vi "ukol1.vi"() -> ()   [LabVIEW 2023]
uses:
  <vilib>/Analysis/2dsp.llb/1D Convolution (DBL).vi
  <vilib>/Analysis/NI_AALPro.lvlib
panel:
  in  "Array 7":dbl[](array[numeric])
  in  "Array 6":dbl[](array[numeric])
  out "Waveform Graph":dbl[][](graph)
  in  "Array 4":dbl[](array[numeric])
  in  "Array 3":dbl[](array[numeric])
  out "X * Y":dbl[](array[numeric])
  out "Array 2":dbl[](array[numeric])
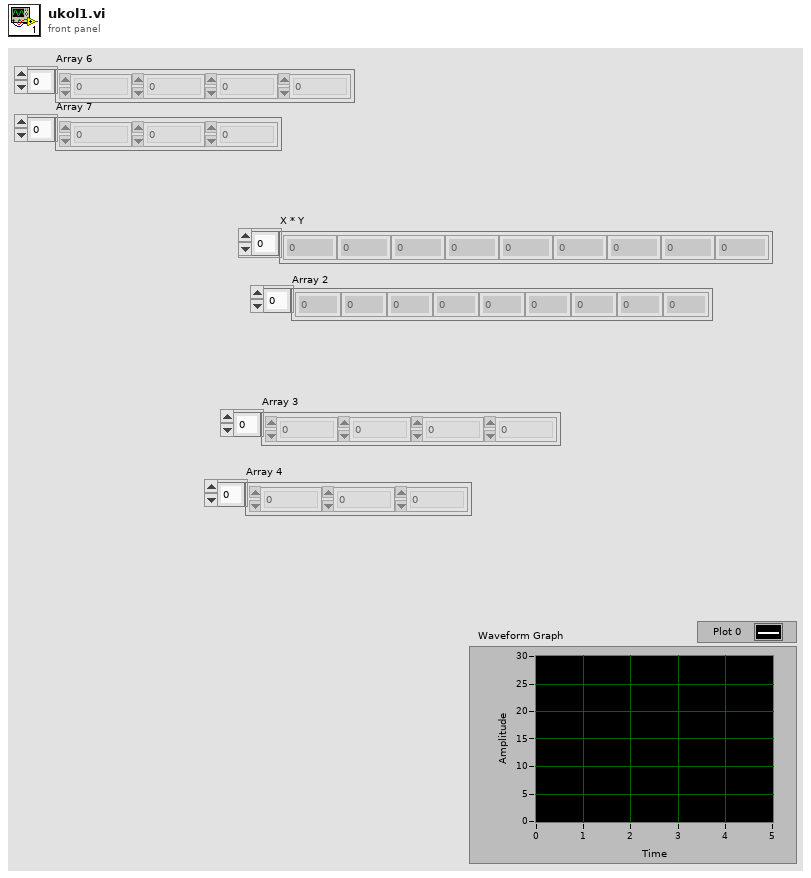
[diagram p1: front panel]
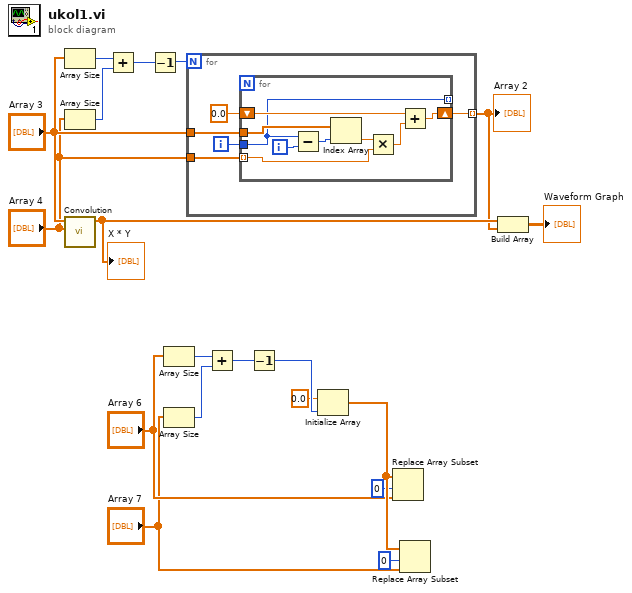
[diagram p0: block diagram]
diagram:
  n1 = Array Size(array="Array 3") -> (size(s)=w18:i32)
  n2 = Array Size(array="Array 4") -> (size(s)=w17:i32)
  n3 = call-poly <vilib>:"Convolution.vi"("Y"="Array 4", "X"="Array 3") -> ("X * Y"=w13:dbl[])  [unwired: 8 in, 1 out]
  "X * Y" <- w13
  n4 = Add(x=w18, y=w17) -> (x+y=w19:i32)
  n5 = Decrement(x=w19) -> (x-1=w16:i32)
  n6 = Array Size(array="Array 6") -> (size(s)=w9:i32)
  n7 = Array Size(array="Array 7") -> (size(s)=w8:i32)
  n8 = for {
    N: w16 -> [_]
    tunnel: "Array 3" -> [w20]
    tunnel: "Array 4" -> [w23]
    tunnel: [w22] -> w12 mode=indexing
    i -> [w21]
    n9 = for {
      shift-right: [w31] -> w22
      shift-left: 0.0 -> [w32]
      tunnel: w23 -> [w30] mode=indexing
      tunnel: w21 -> [w25]
      tunnel: w20 -> [w28]
      tunnel: [w25] -> _ mode=indexing
      i -> [w29]
      n10 = Subtract(x=w25, y=w29) -> (x-y=w27:i32)
      n11 = Index Array(array=w28, index=w27) -> (element=w26:dbl)
      n12 = Multiply(x=w26, y=w30) -> (x*y=w33:dbl)
      n13 = Add(x=w32, y=w33) -> (x+y=w31:dbl)
    }
  }
  "Array 2" <- w12
  n14 = Add(x=w9, y=w8) -> (x+y=w10:i32)
  n15 = Decrement(x=w10) -> (x-1=w7:i32)
  n16 = Initialize Array(0.0 ("element"), w7) -> (w5:dbl[])
  n17 = Replace Array Subset(array=w5, new element="Array 6", index=0) -> ()  [unwired: 1 out]
  n18 = Replace Array Subset(array=w5, new element="Array 7", index=0) -> ()  [unwired: 1 out]
  n19 = Build Array(w13, w12) -> (→"Waveform Graph":dbl[][])
